vi "Queued Message Handler.vi"() -> ()   [LabVIEW 2026]
doc: "Demonstrates the fundamentals of the Queued Message Handler design pattern in LabVIEW. A queued message handler, in its simplest form, is composed of two loops. The Event Handling Loop responds to user interface events by enqueuing \"messages\" on a message queue. These messages are dequeued in the Message Handling Loop. Note that the Message Handling Loop is also capable of sending messages to itself."
uses:
  Program Files/National Instruments/LabVIEW 2026/examples/Design Patterns/Queued Message Handler/support/QMH Fundamentals - Message Cluster.ctl
  <vilib>/Utility/error.llb/Error Cluster From Error Code.vi
  <vilib>/ErrorRing/Error Ring.xnode
panel:
  out "Display Message":string
  in  "Action 2":bool
  in  "Action 1":bool
  in  "Stop":bool
  # "Overview: Demonstrates the fundamental concepts of the Queued Message Handler design pattern in LabVIEW.\nInstructions:\n1. Run the VI.\n2. Click the Action 1 button. The Display Message indicator is updated.\n3. Click the Action 2 button. The Display Message indicator is updated again.\n4. Click Stop to stop the VI."
  # "Note: If you are creating a LabVIEW application based on the Queued Message Handler design pattern, create a Queued Message Handler project from the File > Create Project dialog."
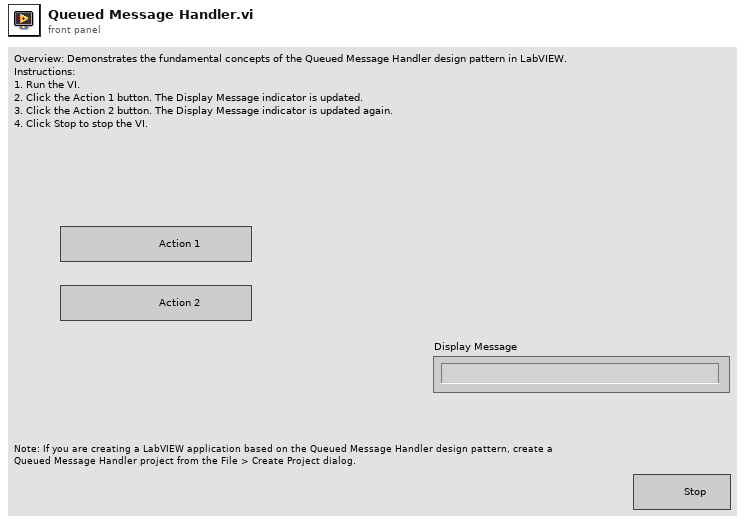
[diagram p1: front panel]
types:
  T1 = typedef "QMH Fundamentals - Message Cluster.ctl" = cluster{"Message":string, "Message Data":variant}
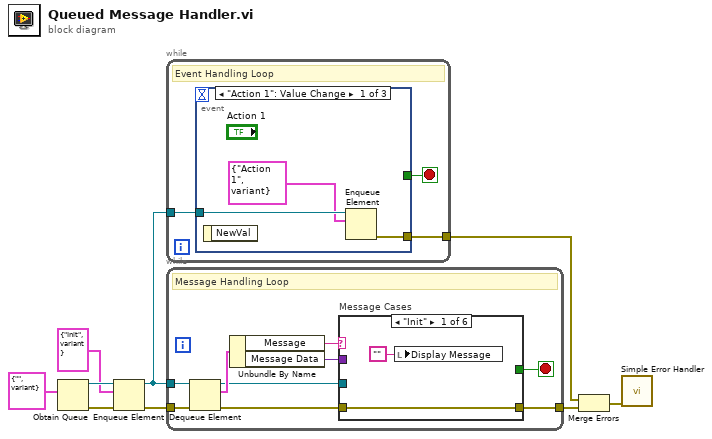
[diagram p0: block diagram]
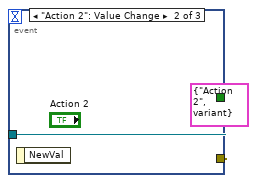
[diagram p2: hidden frame]
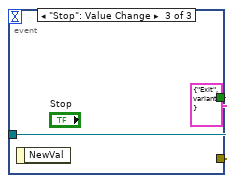
[diagram p3: hidden frame]
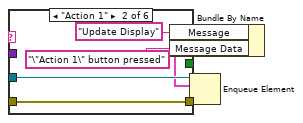
[diagram p4: hidden frame]
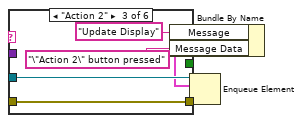
[diagram p5: hidden frame]
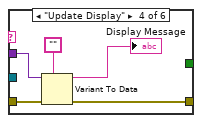
[diagram p6: hidden frame]
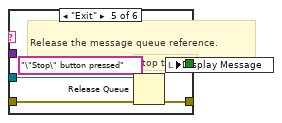
[diagram p7: hidden frame]
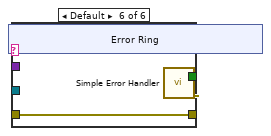
[diagram p8: hidden frame]
diagram:
  n1 = Obtain Queue(element data type=T1 {"Message"="", "Message Data"=variant} ("Message Cluster")) -> (queue out=w5:refnum<queue>, error out=w6:errorcluster)  [unwired: 4 in, 1 out]
  n2 = Enqueue Element(queue=w5, element=T1 {"Message"="Init", "Message Data"=variant}, error in (no error)=w6) -> (queue out=w3:refnum<queue>, error out=w4:errorcluster)  [unwired: 1 in, 1 out]
  n3 = while {
    tunnel: w3 -> [w12]
    tunnel: [w10] -> w8
    stop <- w11 stop-if-true
    # "Event Handling Loop"
    n4 = event shown="[0] \"Action 1\": Value Change" {
      selector: _ -> [_ _ _]
      dyn-events: _ -> [_ _ _]
      timeout: _ -> [_ _ _]
      tunnel: [_ _ TRUE] -> w11
      tunnel: w12 -> [w15 w18 w22]
      tunnel: [w14 w17 w21] -> w10
      event "Action 1": Value Change {
        # "Enqueue an \"Action 1\" message."
        n5 = event-data() -> ()  [unwired: 1 in, 1 out]
        n6 = Enqueue Element(queue=w15, element=T1 {"Message"="Action 1", "Message Data"=variant}) -> (error out=w14:errorcluster)  [unwired: 2 in, 2 out]
      }
      event "Action 2": Value Change {
        # "Enqueue an \"Action 2\" message."
        n7 = event-data() -> ()  [unwired: 1 in, 1 out]
        n8 = Enqueue Element(queue=w18, element=T1 {"Message"="Action 2", "Message Data"=variant}) -> (error out=w17:errorcluster)  [unwired: 2 in, 2 out]
      }
      event "Stop": Value Change {
        # "Stop the VI."
        # "Enqueue an \"Exit\" message. Note that the Enqueue Element At Opposite End function is used to place this priority \"Exit\" message at the front of the queue ahead of all other messages."
        n9 = event-data() -> ()  [unwired: 1 in, 1 out]
        n10 = Enqueue Element At Opposite End(queue=w22, element=T1 {"Message"="Exit", "Message Data"=variant}) -> (error out=w21:errorcluster)  [unwired: 2 in, 2 out]
      }
    }
  }
  n11 = while {
    tunnel: w3 -> [w28]
    tunnel: w4 -> [w29]
    tunnel: [w30] -> w9
    stop <- w31 stop-if-true
    # "Message Handling Loop"
    n12 = Dequeue Element(queue=w28, error in (no error)=w29) -> (queue out=w26:refnum<queue>, element=w27:T1, error out=w25:errorcluster)  [unwired: 1 in, 1 out]
    n13 = Unbundle By Name(w27) -> ("Message"=w24:string, "Message Data"=w23:variant)
    n14 = case "Message Cases" shown="\"Init\"" w24 {
      selector: w24 -> [_ _ _ _ _ w60]
      tunnel: w26 -> [_ w40 w47 _ w57 _]
      tunnel: w25 -> [w33 w38 w45 w52 w54 w59]
      tunnel: [w33 w39 w46 w49 w55 w59] -> w30
      tunnel: [_ _ _ _ TRUE _] -> w31
      tunnel: w23 -> [_ _ _ w51 _ _]
      frame "Init" {
        # "Initialize - Perform any initialization code for your application here. In this example, the only initialization required is setting the Display Message indicator value to an empty string."
        n15 = local write "Display Message"("") -> ()
      }
      frame "Action 1" {
        # "Action 1 - Send an \"Update Display\" message indicating which button was pressed. Note that a string is sent as the Message Data along with the \"Update Display\" message."
        n16 = Bundle By Name(cluster=T1 {"Message"="", "Message Data"=variant} ("Message Cluster"), "Message"="Update Display", "Message Data"="\"Action 1\" button pressed" ("L10n_Action 1 Pressed")) -> (w35:T1)
        n17 = Enqueue Element(queue=w40, element=w35, error in (no error)=w38) -> (error out=w39:errorcluster)  [unwired: 1 in, 2 out]
      }
      frame "Action 2" {
        # "Action 2 - Send an \"Update Display\" message indicating which button was pressed. Note that a string is sent as the Message Data along with the \"Update Display\" message."
        n18 = Bundle By Name(cluster=T1 {"Message"="", "Message Data"=variant} ("Message Cluster"), "Message"="Update Display", "Message Data"="\"Action 2\" button pressed" ("L10n_Action 2 Pressed")) -> (w42:T1)
        n19 = Enqueue Element(queue=w47, element=w42, error in (no error)=w45) -> (error out=w46:errorcluster)  [unwired: 1 in, 2 out]
      }
      frame "Update Display" {
        # "Update Display - Convert the Message Data to a string to display in the Display Message indicator."
        n20 = Variant To Data(error in=w52, type="", Variant=w51) -> (data=→"Display Message":string, error out=w49:errorcluster)
      }
      frame "Exit" {
        # "Stop the VI."
        # "Release the message queue reference."
        # "Exit - Exit the application. Since this message was sent as a priority message (i.e., it was placed at the front of the queue), any cleanup code should run here, since the loop is about to stop. Any other messages in the queue will not be handled."
        n21 = Release Queue(queue=w57, error in (no error)=w54) -> (error out=w55:errorcluster)  [unwired: 1 in, 2 out]
        n22 = local write "Display Message"("\"Stop\" button pressed" ("L10n_Stop Pressed")) -> ()
      }
      frame Default {
        # "The Default case only runs if there is a message that isn't defined in any of the other cases. Generate an error if this occurs."
        n23 = xnode "Error Ring"("parameter 0"=w60) -> ("error out"=w58:errorcluster)
        n24 = call <vilib>:"Simple Error Handler.vi"("error in (no error)"=w58) -> ()  [unwired: 4 in, 5 out]
      }
    }
  }
  n25 = Merge Errors(w8, w9) -> (w1:errorcluster)
  n26 = call <vilib>:"Simple Error Handler.vi"("error in (no error)"=w1) -> ()  [unwired: 4 in, 5 out]
